vi "例4-12.vi"() -> ()   [LabVIEW 2019]
panel:
  out "数组3":dbl[](array[numeric])
  in  "数组2":dbl[](array[numeric])
  in  "数值2":dbl=5.0
  in  "数值1":dbl=4.0
  in  "数组1":dbl[](array[numeric])
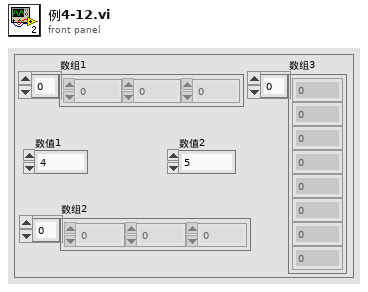
[diagram p1: front panel]
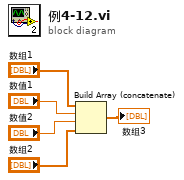
[diagram p0: block diagram]
diagram:
  n1 = Build Array (concatenate)("数组1", "数值1", "数值2", "数组2") -> (→"数组3":dbl[])
